vi "16ChannelRecorderv2.vi"() -> ()   [LabVIEW 2013]
doc: "Cont(inuous) Acq(uire) & Chart (hw timed) demonstrates the hardware timed, non-buffered technique of data acquisition. The scan clock on the board controls acquisition timing. Acquired scans are read directly from the device's FIFO using AI Single Scan. \n\nThe acquisition is configured with no buffer, and the on-board scan clock started at the selected scan rate. In the first loop iteration, the newest (most recent) scan is read from the FIFO. In each subsequent loop iteration AI Single Scan is called to read the oldest scan from the FIFO. Then if a scan is missed because the acquisition does not keep up, an error message will be displayed, and the acquisition stopped. Each scan is plotted on the chart after it is read. \n\nA common reason to use non-buffered acquisition is that some kind of processing needs to be done for each data point. You will probably want to add more functions to the diagram to customize this VI for your application. The acquisition rate you can achieve depends on how much processing and display the VI must do. This VI calls a subVI named My Single-Scan Processing. Add whatever processing you need to this subVI, or replace it with one of your own. The data processing subVI also demonstrates how to use error clusters in your own subVIs, so they can be included in the error data flow chain.\n\nBefore running this VI, set the values of the controls on the front panel. Select Show Help Window from the Help menu to see a description of each control. If the values you select for all the controls are values you will usually use, select Make Current Values Default from the Operate menu and save the VI. Or, you may save individual control's default values by popping up on the control, selecting Data Operations, then selecting Make Current Value Default, and saving the VI."
uses:
  <vilib>/Utility/error.llb/DialogType.ctl
  <vilib>/DAQmx/read.llb/DAQmx Read (Analog 2D DBL NChan NSamp).vi
  BiaxGlobals (16chan).vi
  <vilib>/DAQmx/create/channels.llb/DAQmx Create Channel (AI-Voltage-Basic).vi
  <vilib>/DAQmx/configure/timing.llb/DAQmx Timing (Sample Clock).vi
  effectiveglobals.vi
  <vilib>/DAQmx/miscellaneous.llb/DAQmx Fill In Error Info.vi
panel:
  in  "Show plot":bool
  out "Zero Voltage Y":dbl
  in  "Calibration y-axis (V/unit)":dbl=1.0 format="%#_6f"
  in  "Select y-axis":string(combo)="Porosity"
  in  "Calibration x-axis (V/unit)":dbl=1.0 format="%#_6f"
  in  "Select x-axis":string(combo)="Time (s)"
  out "Offset Voltage 2":dbl
  out "Offset Voltage 1":dbl
  in  "Offset X-axis 2":bool
  in  "Offset X-axis 1":bool
  in  "Zero y-axis":bool
  out "XY plot":cluster{"Y":dbl[], "Y":dbl[]}[](graph)
  in  "Reset plot":bool
  out "Zero Voltage X":dbl
  in  "Zero X-axis":bool
  out "Porosity (%)":dbl format="%_4f"
  in  "Material density (g/cm3)":dbl=2.17
  in  "Amount of material (g)":dbl=42.88 format="%_4f"
  in  "Thickness (2 layers, mm)":dbl=11.28 format="%_4f"
  in  "Zero Hor DCDT":bool
  out "Average Pore pressure":dbl=0.0015205308
  out "Zeroed at:":i32
  out "Zero Voltage":dbl format="%_6g"
  in  "Zero Pore pressure A":bool
  out "Zeroed at:":i32
  out "Zero Voltage":dbl format="%_6g"
  in  "Zero Pore pressure B":bool
  out "Effective normal \nstress (MPa)":dbl=0.0015205308
  in  "Sample\n Area (m2)":dbl=0.003078
  out "Zeroed at:":i32
  out "Zero Voltage":dbl format="%_6g"
  in  "Zero Confine":bool
  in  "Horizontal Load":bool=TRUE
  out "Zeroed at:":i32
  out "Zero Voltage":dbl format="%_6g"
  in  "Zero Normal":bool
  out "Array 2":i32[][](array[numeric])=[[10000, 0, -17, -1030, -696, -422, -1063, -1097, -410, -661, -1080]]
  out "AUX8 (ch11)":dbl format="%.4f"
  out "AUX7 (ch10)":dbl format="%.4f"
  out "AUX6 (ch9)":dbl format="%.4f"
  out "AUX5 (ch8)":dbl format="%.4f"
  out "AUX4 (ch7)":dbl format="%.4f"
  out "AUX3 (ch6)":dbl format="%.4f"
  out "AUX2 (ch5)":dbl format="%.4f"
  out "AUX1 (ch4)":dbl format="%.4f"
  out "Hor Load (ch0)":dbl format="%.4f"
  out "Vert Load (ch2)":dbl format="%.4f"
  out "Hor LVDT":dbl format="%.4f"
  out "Vert LVDT (ch3)":dbl format="%.4f"
  out "Array 17":i32[][](array[numeric])=[[10000, -673, -5, -1015, -683, -421, -1049, -1100, -413, -693, -1121]]
  out "Array 16":i32[][](array[numeric])=[[10000, -673, -5, -1015, -683, -421, -1049, -1100, -413, -693, -1121]]
  out "Array 15":i32[][](array[numeric])=[[10000, -673, -5, -1015, -683, -421, -1049, -1100, -413, -693, -1121]]
  out "Array 14":i32[][](array[numeric])=[[10000, -685, -5, -1012, -680, -418, -1052, -1092, -421, -673, -1097]]
  out "AUX12 (ch15)":dbl format="%.4f"
  out "AUX11 (ch14)":dbl format="%.4f"
  out "AUX10 (ch13)":dbl format="%.4f"
  out "AUX9 (ch12)":dbl format="%.4f"
  out "element 15":string
  out "element 14":string
  out "element 13":string
  out "element 12":string
  out "element 11":string
  out "element 10":string
  out "element 9":string
  out "element 8":string
  out "element 7":string
  out "element 6":string="  "
  out "element 5":string
  out "element 4":string
  out "element 3":string
  out "element 2":string
  out "element":string
  out "element":string
  out "Stress-strain-temp vs time (Voltage)":dbl[][](graph)
  out "Array 13":i32[][](array[numeric])
  out "Array 12":i32[][](array[numeric])
  out "Array 11":i32[][](array[numeric])
  out "Array 10":i32[][](array[numeric])
  out "Array 9":i32[][](array[numeric])
  out "Array 8":i32[][](array[numeric])
  out "Array 7":i32[][](array[numeric])
  out "Array 6":i32[][](array[numeric])
  out "Array 5":i32[][](array[numeric])
  out "Array 4":i32[][](array[numeric])
  out "Array 3":i32[][](array[numeric])
  out "Array":i32[][](array[numeric])
  out "10000":bool
  in  "10 kHz":bool
  out "Processor scan rate":i32
  out "Present sample number":i32
  in  "1 Hz":bool
  out "1":bool
  out "10":bool
  out "100":bool
  out "1000":bool
  in  "10 Hz":bool
  in  "100 Hz":bool
  in  "1000 Hz":bool
  out "Data Recording Rate":i32(slide) scale=1.0..10000.0
  out "Write interval":i32
  out "Write countdown":i32
  out "Time into data acq. (s)":i32
  out "Saved sample No.":i32
  out "Record rate (samp/s)":i32
  out "No. of scans in backlog":i32
  in  "stop":bool
  # "To File (24 bit)"
  # "Input Signals (volts)"
  # "S\nI\nG\nN\nA\nL\n\nV\nO\nL\nT\nA\nG\nE"
  # "Timestamp"
  # "Data Recording Info"
  # "Sample (point) Number"
  # "Acquisition Statistics"
  # "Low gain"
  # "High gain"
  # "NOTE:  This instrument will write data (time channel then Channels 0-15) to a user defined filename.  The file is written in binary format without a header. The time channel is comprised of numbers indicating the data recording frequency (eg 1, 10, 100, 1000, 10000  samples per second)."
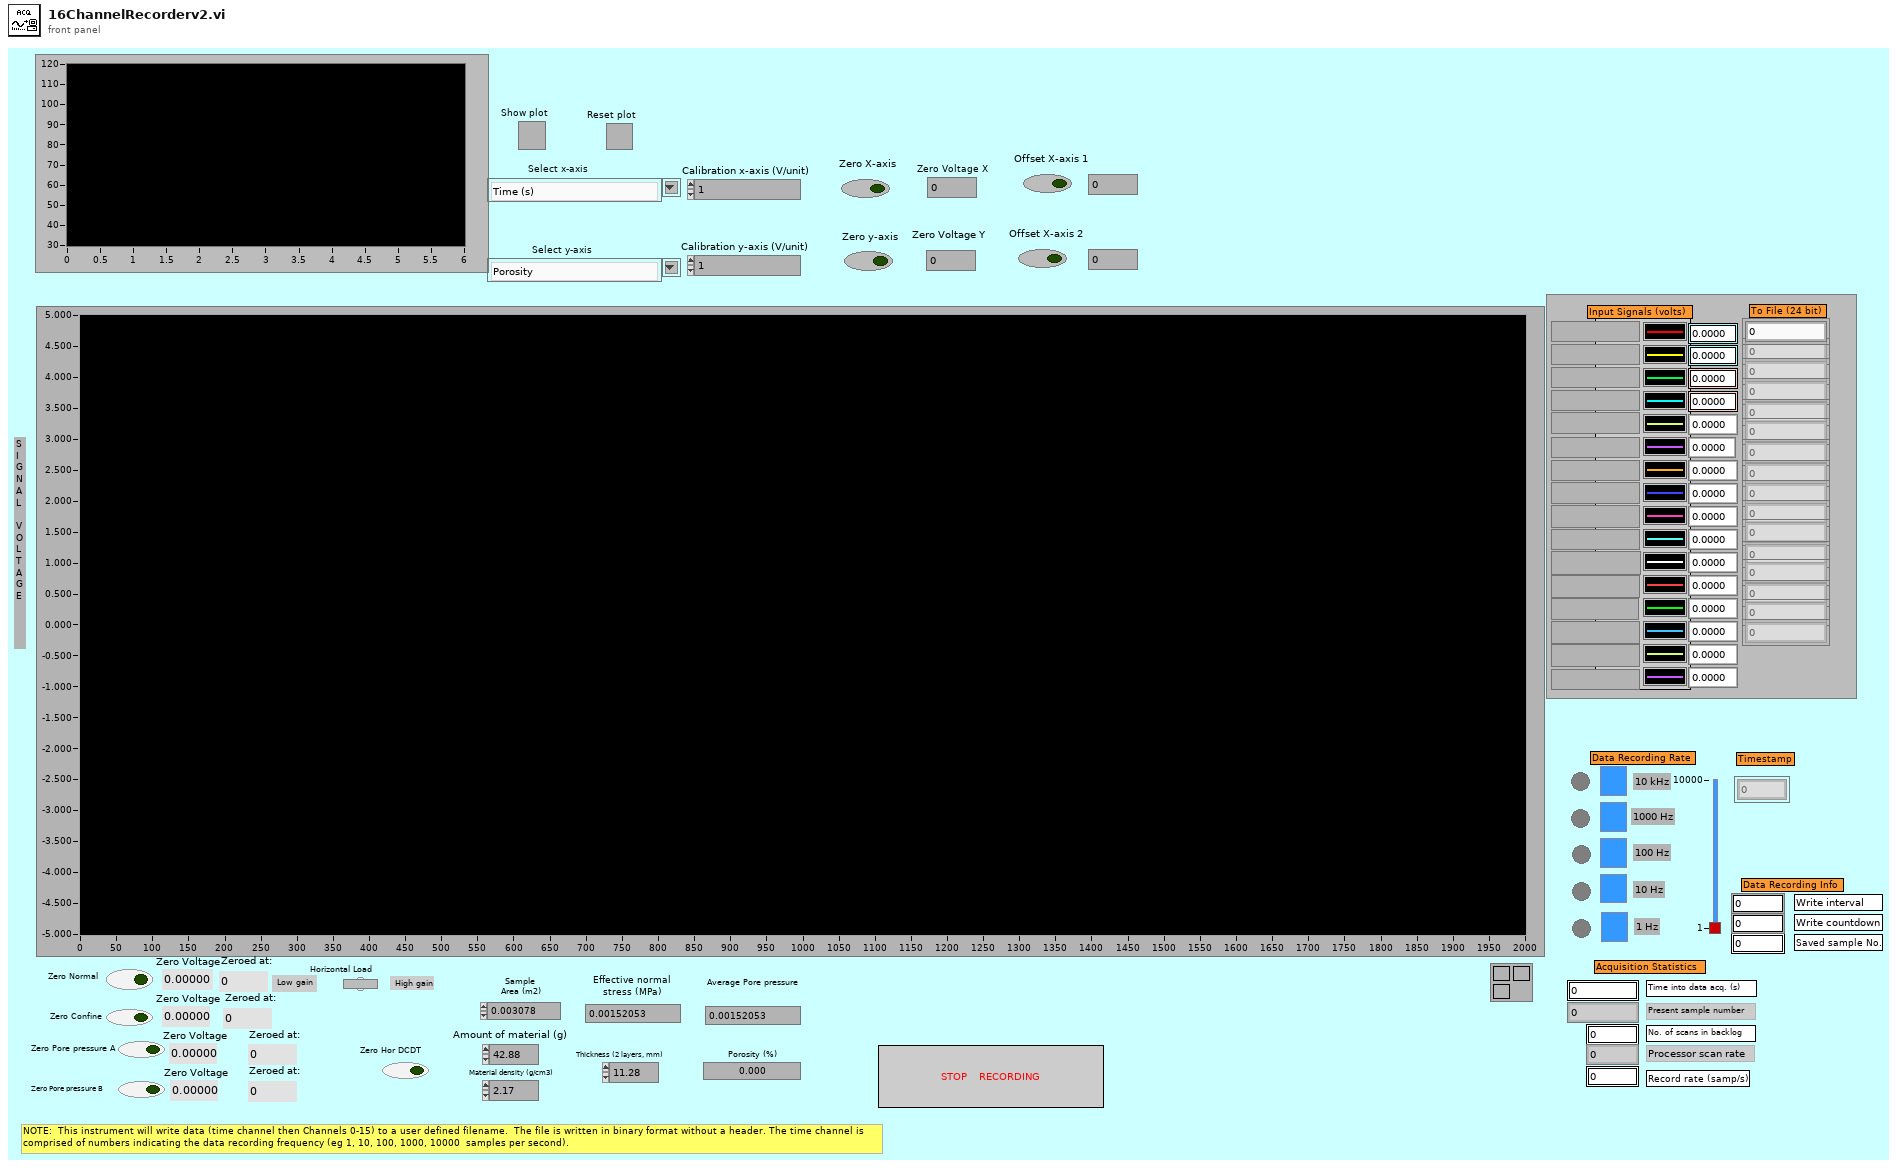
[diagram p1: front panel]
types:
  T1 = typedef "DialogType.ctl" = u16
  T2 = enum16{"big-endian, network order", "native, host order", "little-endian"}
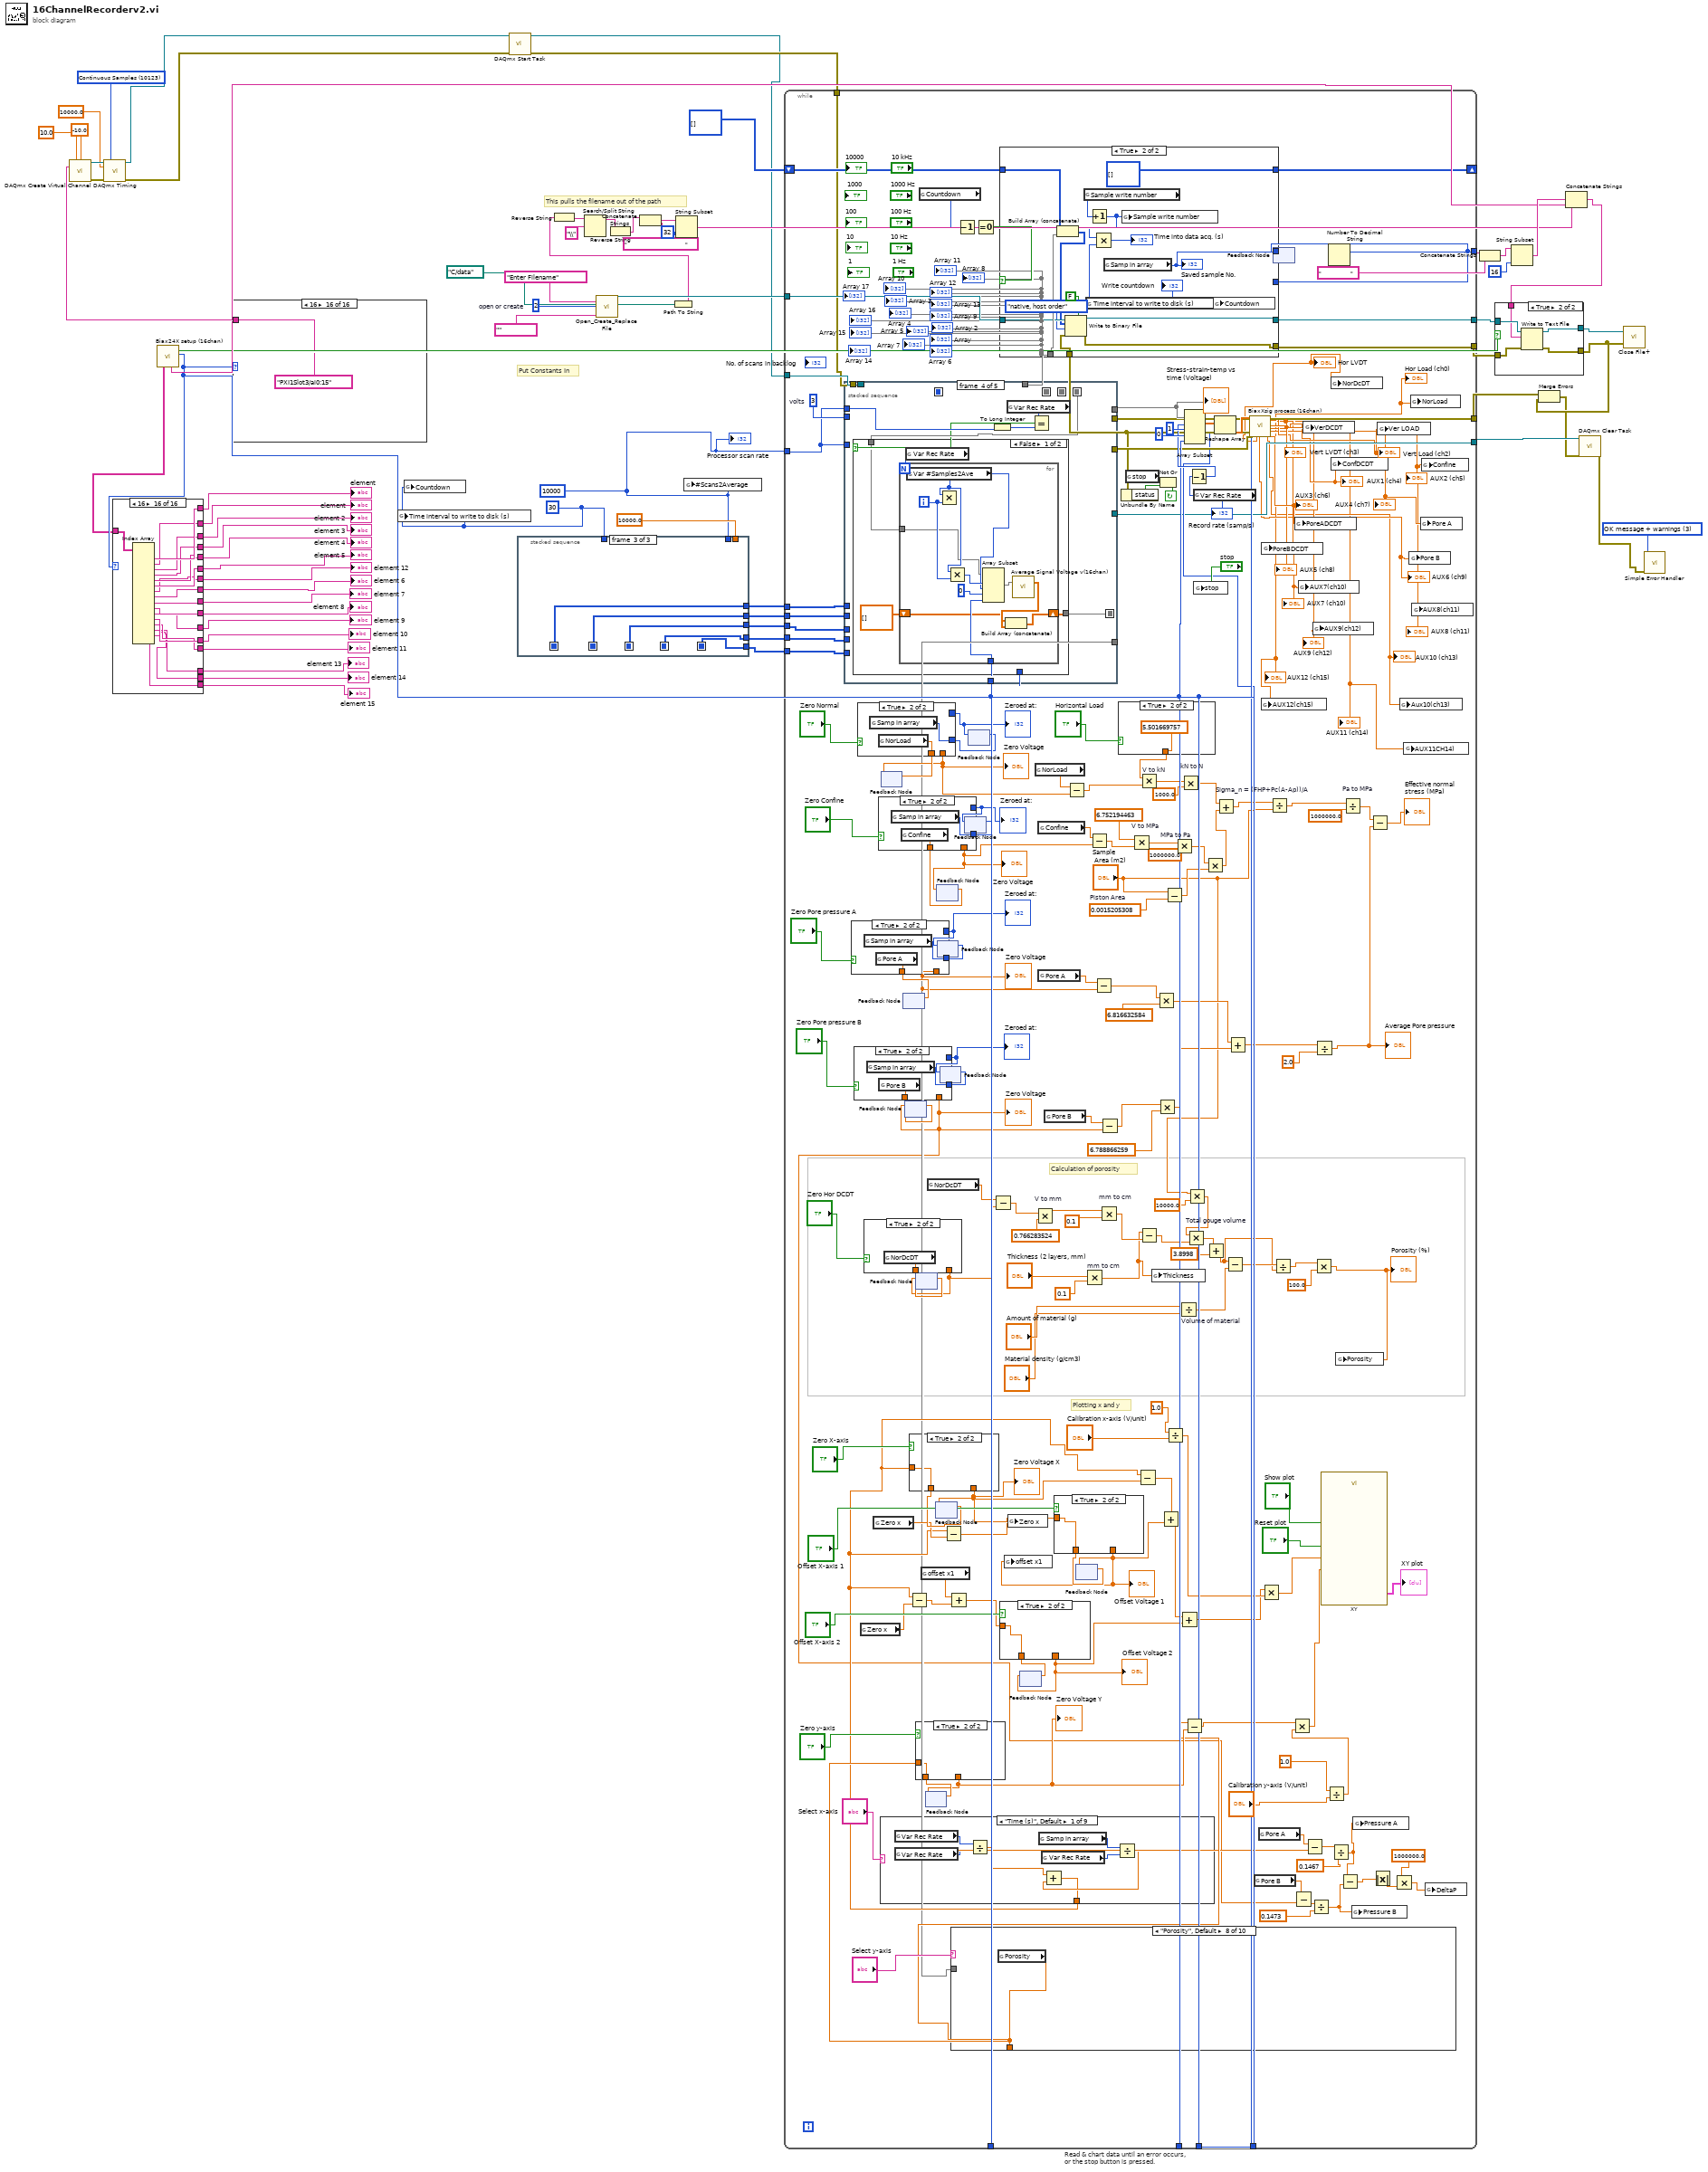
[diagram p0: block diagram]
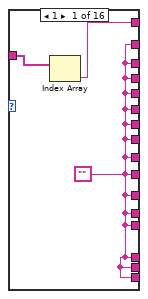
[diagram p2: hidden frame]
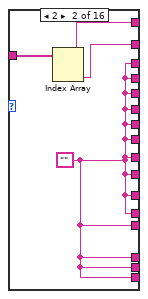
[diagram p3: hidden frame]
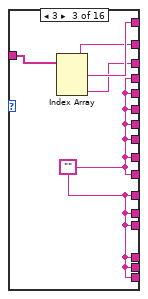
[diagram p4: hidden frame]
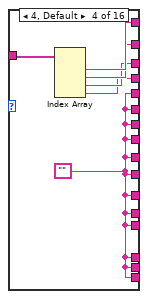
[diagram p5: hidden frame]
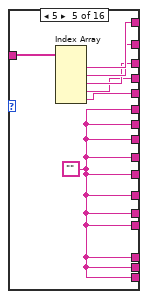
[diagram p6: hidden frame]
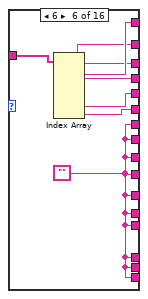
[diagram p7: hidden frame]
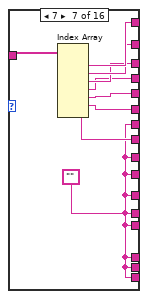
[diagram p8: hidden frame]
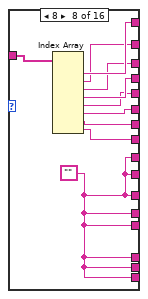
[diagram p9: hidden frame]
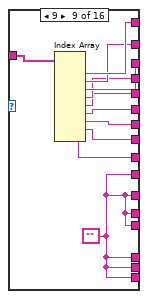
[diagram p10: hidden frame]
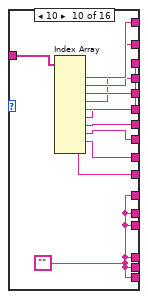
[diagram p11: hidden frame]
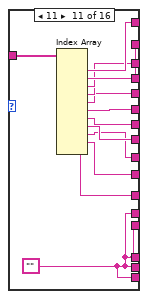
[diagram p12: hidden frame]
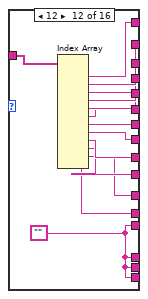
[diagram p13: hidden frame]
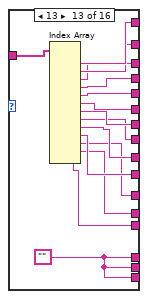
[diagram p14: hidden frame]
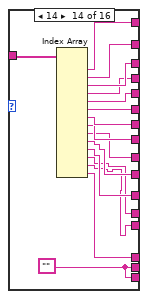
[diagram p15: hidden frame]
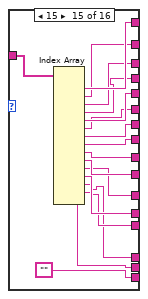
[diagram p16: hidden frame]
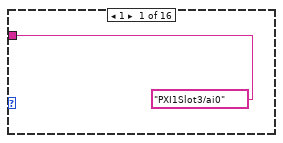
[diagram p18: hidden frame]
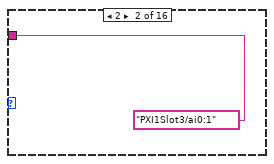
[diagram p19: hidden frame]
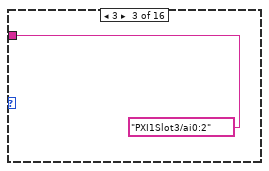
[diagram p20: hidden frame]
diagram:
  w11 = T1 3 items=["no dialog", "OK message", "continue or stop message", "OK message + warnings", "continue/stop + warnings"] ("type of dialog (OK msg:1)")
  w12 = 10000 ("Number of scans")
  w47 = 30 ("Write time int (s)")
  w50 = 10123 items=["Finite Samples"=10178, "Continuous Samples"=10123, "Hardware Timed Single Point"=12522] ("sample mode")
  w71 = 2  # open or create
  # "This pulls the filename out of the path"
  # "Put Constants In"
  n1 = call "Biax24X setup (16chan).vi"() -> ("Footer String"=w36:string, "Number of Channels"=w30:i32, "ASCII footer 2"=w35:bool, "Channel Names"=w29:string[])  [unwired: 1 in, 4 out]
  n2 = case shown="16" w30 {
    tunnel: w29 -> [w74 w77 w82 w88 w95 w103 w112 w123 w134 w146 w159 w173 w188 w202 w219 w238]
    tunnel: [w73 w78 w83 w89 w96 w104 w113 w122 w133 w145 w158 w172 w187 w201 w220 w237] -> w18
    tunnel: [w72 w76 w81 w87 w94 w102 w111 w121 w132 w144 w157 w171 w186 w200 w218 w236] -> w28
    tunnel: [w72 w75 w80 w86 w93 w101 w110 w120 w131 w143 w156 w170 w185 w199 w217 w235] -> w27
    tunnel: [w72 w75 w79 w85 w92 w100 w109 w119 w130 w142 w155 w169 w184 w198 w216 w234] -> w26
    tunnel: [w72 w75 w79 w84 w91 w99 w108 w118 w129 w141 w154 w168 w183 w197 w215 w233] -> w25
    tunnel: [w72 w75 w79 w84 w90 w98 w107 w117 w128 w140 w153 w167 w182 w196 w214 w232] -> w24
    tunnel: [w72 w75 w79 w84 w90 w97 w106 w115 w126 w138 w151 w165 w180 w194 w212 w230] -> w23
    tunnel: [w72 w75 w79 w84 w90 w97 w105 w114 w125 w137 w150 w164 w179 w193 w211 w229] -> w22
    tunnel: [w72 w75 w79 w84 w90 w97 w105 w114 w124 w136 w149 w163 w178 w191 w210 w228] -> w21
    tunnel: [w72 w75 w79 w84 w90 w97 w105 w114 w124 w135 w148 w162 w177 w192 w209 w227] -> w20
    tunnel: [w72 w75 w79 w84 w90 w97 w105 w114 w124 w135 w147 w161 w176 w190 w208 w226] -> w19
    tunnel: [w72 w75 w79 w84 w90 w97 w105 w114 w124 w135 w147 w160 w175 w189 w207 w225] -> w17
    tunnel: [w72 w75 w79 w84 w90 w97 w105 w114 w124 w135 w147 w160 w174 w203 w206 w224] -> w16
    tunnel: [w72 w75 w79 w84 w90 w97 w105 w114 w124 w135 w147 w160 w174 w204 w205 w223] -> w15
    tunnel: [w72 w75 w79 w84 w90 w97 w105 w114 w124 w135 w147 w160 w174 w204 "" w222] -> w14
    tunnel: [w72 w75 w79 w84 w90 w97 w105 w116 w127 w139 w152 w166 w181 w195 w213 w231] -> w13
    frame 1 {
      w72 = ""
      n3 = Index Array(array=w74) -> (element=w73:string)  [unwired: 1 in]
    }
    frame 2 {
      w75 = ""
      n4 = Index Array(array=w77) -> (element #1=w78:string, element #2=w76:string)  [unwired: 2 in]
    }
    frame 3 {
      w79 = ""
      n5 = Index Array(array=w82) -> (element #1=w83:string, element #2=w81:string, element #3=w80:string)  [unwired: 3 in]
    }
    frame 4, Default {
      w84 = ""
      n6 = Index Array(array=w88) -> (element #1=w89:string, element #2=w87:string, element #3=w86:string, element #4=w85:string)  [unwired: 4 in]
    }
    frame 5 {
      w90 = ""
      n7 = Index Array(array=w95) -> (element #1=w96:string, element #2=w94:string, element #3=w93:string, element #4=w92:string, element #5=w91:string)  [unwired: 5 in]
    }
    frame 6 {
      w97 = ""
      n8 = Index Array(array=w103) -> (element #1=w104:string, element #2=w102:string, element #3=w101:string, element #4=w100:string, element #5=w99:string, element #6=w98:string)  [unwired: 6 in]
    }
    frame 7 {
      w105 = ""
      n9 = Index Array(array=w112) -> (element #1=w113:string, element #2=w111:string, element #3=w110:string, element #4=w109:string, element #5=w108:string, element #6=w107:string, element #7=w106:string)  [unwired: 7 in]
    }
    frame 8 {
      w114 = ""
      n10 = Index Array(array=w123) -> (element #1=w122:string, element #2=w121:string, element #3=w120:string, element #4=w119:string, element #5=w118:string, element #6=w117:string, element #7=w116:string, element #8=w115:string)  [unwired: 8 in]
    }
    frame 9 {
      w124 = ""
      n11 = Index Array(array=w134) -> (element #1=w133:string, element #2=w132:string, element #3=w131:string, element #4=w130:string, element #5=w129:string, element #6=w128:string, element #7=w127:string, element #8=w126:string, element #9=w125:string)  [unwired: 9 in]
    }
    frame 10 {
      w135 = ""
      n12 = Index Array(array=w146) -> (element #1=w145:string, element #2=w144:string, element #3=w143:string, element #4=w142:string, element #5=w141:string, element #6=w140:string, element #7=w139:string, element #8=w138:string, element #9=w137:string, element #10=w136:string)  [unwired: 10 in]
    }
    frame 11 {
      w147 = ""
      n13 = Index Array(array=w159) -> (element #1=w158:string, element #2=w157:string, element #3=w156:string, element #4=w155:string, element #5=w154:string, element #6=w153:string, element #7=w152:string, element #8=w151:string, element #9=w150:string, element #10=w149:string, element #11=w148:string)  [unwired: 11 in]
    }
    frame 12 {
      w160 = ""
      n14 = Index Array(array=w173) -> (element #1=w172:string, element #2=w171:string, element #3=w170:string, element #4=w169:string, element #5=w168:string, element #6=w167:string, element #7=w166:string, element #8=w165:string, element #9=w164:string, element #10=w163:string, element #11=w162:string, element #12=w161:string)  [unwired: 12 in]
    }
    frame 13 {
      w174 = ""
      n15 = Index Array(array=w188) -> (element #1=w187:string, element #2=w186:string, element #3=w185:string, element #4=w184:string, element #5=w183:string, element #6=w182:string, element #7=w181:string, element #8=w180:string, element #9=w179:string, element #10=w178:string, element #11=w177:string, element #12=w176:string, element #13=w175:string)  [unwired: 13 in]
    }
    frame 14 {
      w204 = ""
      n16 = Index Array(array=w202) -> (element #1=w201:string, element #2=w200:string, element #3=w199:string, element #4=w198:string, element #5=w197:string, element #6=w196:string, element #7=w195:string, element #8=w194:string, element #9=w193:string, element #10=w191:string, element #11=w192:string, element #12=w190:string, element #13=w189:string, element #14=w203:string)  [unwired: 14 in]
    }
    frame 15 {
      n17 = Index Array(array=w219) -> (element #1=w220:string, element #2=w218:string, element #3=w217:string, element #4=w216:string, element #5=w215:string, element #6=w214:string, element #7=w213:string, element #8=w212:string, element #9=w211:string, element #10=w210:string, element #11=w209:string, element #12=w208:string, element #13=w207:string, element #14=w206:string, element #15=w205:string)  [unwired: 15 in]
    }
    frame 16 {
      n18 = Index Array(array=w238) -> (element #1=w237:string, element #2=w236:string, element #3=w235:string, element #4=w234:string, element #5=w233:string, element #6=w232:string, element #7=w231:string, element #8=w230:string, element #9=w229:string, element #10=w228:string, element #11=w227:string, element #12=w226:string, element #13=w225:string, element #14=w224:string, element #15=w223:string, element #16=w222:string)  [unwired: 16 in]
    }
  }
  "element" <- w18
  "element" <- w28
  "element 2" <- w27
  "element 3" <- w26
  "element 4" <- w25
  "element 5" <- w24
  "element 6" <- w23
  "element 7" <- w22
  "element 8" <- w21
  "element 9" <- w20
  "element 10" <- w19
  "element 11" <- w17
  "element 12" <- w13
  "element 13" <- w16
  "element 14" <- w15
  "element 15" <- w14
  n19 = case shown="16" w30 {
    tunnel: [tag "PXI1Slot3/ai0" ("physical channels") tag "PXI1Slot3/ai0:1" ("physical channels") tag "PXI1Slot3/ai0:2" ("physical channels") tag "PXI1Slot3/ai0:3" ("physical channels") tag "PXI1Slot3/ai0:4" ("physical channels") tag "PXI1Slot3/ai0:5" ("physical channels") tag "PXI1Slot3/ai0:6" ("physical channels") tag "PXI1Slot3/ai0:7" ("physical channels") tag "PXI1Slot3/ai0:8" ("physical channels") tag "PXI1Slot3/ai0:9" ("physical channels") tag "PXI1Slot3/ai0:10" ("physical channels") tag "PXI1Slot3/ai0:11" ("physical channels") tag "PXI1Slot3/ai0:12" ("physical channels") tag "PXI1Slot3/ai0:13" ("physical channels") tag "PXI1Slot3/ai0:14" ("physical channels") tag "PXI1Slot3/ai0:15" ("physical channels")] -> w44
    frame 1 {
    }
    frame 2 {
    }
    frame 3 {
    }
    frame 4, Default {
    }
    frame 5 {
    }
    frame 6 {
    }
    frame 7 {
    }
    frame 8 {
    }
    frame 9 {
    }
    frame 10 {
    }
    frame 11 {
    }
    frame 12 {
    }
    frame 13 {
    }
    frame 14 {
    }
    frame 15 {
    }
    frame 16 {
    }
  }
  n20 = call-poly <vilib>:"DAQmx Create Virtual Channel.vi"("maximum value"=10.0, "minimum value"=-10.0, "physical channels"=w44) -> ("task out"=w52:refnum<k21>, "error out"=w51:errorcluster)  [unwired: 11 in]
  n21 = call-poly <vilib>:"DAQmx Timing.vi"("task/channels in"=w52, "sample mode"=w50, "rate"=10000.0, "error in"=w51) -> ("task out"=w5:refnum<k21>, "error out"=w4:errorcluster)  [unwired: 10 in]
  n22 = global write "BiaxGlobals (16chan).vi" "Time interval to write to disk (s)"(w47) -> ()
  n23 = global write "BiaxGlobals (16chan).vi" "Countdown"(w47) -> ()
  n24 = call <vilib>:"DAQmx Start Task.vi"("task/channels in"=w5, "error in"=w4) -> ("task out"=w1:refnum<k21>, "error out"=w2:errorcluster)  [unwired: 12 in]
  n25 = stacked-sequence {
    seq-local: [_ w275 _] -> [_ _ w288]
    seq-local: [_ w272 _] -> [_ _ w285]
    seq-local: [_ w267 _] -> [_ _ w287]
    seq-local: [_ w266 _] -> [_ _ w286]
    seq-local: [_ w261 _] -> [_ _ w284]
    tunnel: w47 -> [w255 _ _]
    tunnel: w12 -> [w259 _ _]
    tunnel: sgl 10000.0 ("actual scan rate") -> [w257 _ _]
    tunnel: [_ _ w288] -> w66
    tunnel: [_ _ w285] -> w65
    tunnel: [_ _ w287] -> w64
    tunnel: [_ _ w286] -> w63
    tunnel: [_ _ w284] -> w62
    frame #0 {
      w256 = i16 0
      n26 = local write "Time into data acq. (s)"(w256) -> ()
      n27 = global write "BiaxGlobals (16chan).vi" "Sample write number"(w256) -> ()
      n28 = global write "BiaxGlobals (16chan).vi" "Time interval to write to disk (s)"(w255) -> ()
      n29 = Divide(x=w257, y=w259) -> (x/y=w258:sgl)
      n30 = global write "BiaxGlobals (16chan).vi" "Rec Rate (samp/s)"(w258) -> ()
      n31 = local write "Write countdown"(w255) -> ()
      n32 = local write "Saved sample No."(w256) -> ()
      n33 = global write "BiaxGlobals (16chan).vi" "Samp in array"(w256) -> ()
    }
    frame #1 {
      n34 = Initialize Array(i16 1, 10000) -> (w275:i16[])
      n35 = global write "BiaxGlobals (16chan).vi" "Rec Rate case"(4) -> ()
      n36 = local write "10"(FALSE) -> ()
      n37 = local write "1"(TRUE) -> ()
      n38 = Initialize Array(i16 10, 1000) -> (w272:i16[])
      n39 = local write "1000"(FALSE) -> ()
      n40 = local write "100"(FALSE) -> ()
      n41 = global read "BiaxGlobals (16chan).vi" "Time interval to write to disk (s)"() -> (→"Write interval":i32)
      n42 = Initialize Array(i16 100, 100) -> (w267:i16[])
      n43 = local write "10000"(FALSE) -> ()
      n44 = Initialize Array(i16 1000, 10) -> (w266:i16[])
      n45 = Initialize Array(i16 10000, 1) -> (w261:i16[])
      n46 = global write "BiaxGlobals (16chan).vi" "Accum Time"(0) -> ()
      n47 = global write "BiaxGlobals (16chan).vi" "Var Rec Rate"(1) -> ()
    }
    frame #2 {
    }
  }
  n48 = call <vilib>:"Open_Create_Replace File.vi"("default name"="", "prompt"="Enter Filename", "function (open:0)"=w71, "start path  (Not A Path)"=path "C:/data") -> ("new file path"=w61:path, "refnum"=w68:refnum<file>)  [unwired: 4 in, 2 out]
  n49 = Path To String(path=w61) -> (string=w58:string)
  n50 = Reverse String(1:w58) -> (0:w59:string)
  n51 = Search/Split String(string=w59, search string/char (-)="\\") -> (substring before match=w57:string)  [unwired: 1 in, 2 out]
  n52 = Reverse String(1:w57) -> (0:w53:string)
  n53 = Concatenate Strings(w53, "                                ") -> (w55:string)
  n54 = String Subset(string=w55, length (rest)=32 ("length (rest)")) -> (substring=w37:string)  [unwired: 1 in]
  n55 = global write "BiaxGlobals (16chan).vi" "#Scans2Average"(w12) -> ()
  n56 = while "Read & chart data until an error occurs,\nor the stop button is pressed." {
    tunnel: w62 -> [w450]
    tunnel: w63 -> [w452]
    tunnel: w64 -> [w453]
    tunnel: w65 -> [w454]
    tunnel: w66 -> [w455]
    shift-left: i16[][] [] -> [w442]
    shift-right: [w468] -> _
    tunnel: w12 -> [w456]
    tunnel: [w469] -> w32
    tunnel: [w470] -> w34
    tunnel: w68 -> [w471]
    tunnel: w30 -> [w449]
    tunnel: w30 -> [w443]
    tunnel: w30 -> [w448]
    tunnel: w30 -> [w444]
    tunnel: [w440] -> w43
    tunnel: w1 -> [w436]
    tunnel: w2 -> [w435]
    tunnel: [w434] -> w9
    tunnel: [w433] -> w10
    stop <- w467 continue-if-true
    w395 = 0.0015205308  # Piston Area
    w462 = 3  # volts
    # "Plotting x and y"
    # "Calculation of porosity"
    n57 = stacked-sequence {
      seq-local: [_ _ w587 _ _] -> [_ _ _ _ w629]
      seq-local: [_ _ _ w605 _] -> [_ _ _ _ w626]
      seq-local: [w551 _ _ _ _] -> [_ w556 _ _ _]
      seq-local: [_ w556 _ _ _] -> [_ _ w585 _ _]
      seq-local: [_ _ w585 _ _] -> [_ _ _ w604 _]
      tunnel: w462 -> [_ _ _ _ _]
      tunnel: w456 -> [_ _ _ w608 _]
      tunnel: [w549 _ _ _ _] -> w446
      tunnel: [_ _ _ _ w626] -> w439
      tunnel: w456 -> [w555 _ _ _ w634]
      tunnel: w455 -> [_ _ w595 _ _]
      tunnel: w454 -> [_ _ w594 _ _]
      tunnel: w453 -> [_ _ w593 _ _]
      tunnel: w452 -> [_ _ w592 _ _]
      tunnel: [_ _ _ _ w628] -> w437
      tunnel: w450 -> [_ _ w586 _ _]
      tunnel: w448 -> [_ _ _ w606 _]
      tunnel: w435 -> [w553 _ _ _ _]
      tunnel: w436 -> [w554 _ _ _ _]
      tunnel: [w549 _ _ _ _] -> w434
      tunnel: [w552 _ _ _ _] -> w433
      tunnel: [_ _ _ _ w626] -> w308
      frame #0 {
        n58 = call-poly <vilib>:"DAQmx Read.vi"("task/channels in"=w554, "number of samples per channel"=w555, "error in"=w553) -> ("task out"=w552:refnum<k21>, "data"=w550:dbl[][], "error out"=w549:errorcluster)  [unwired: 10 in]
        n59 = Transpose 2D Array(2D array=w550) -> (transposed array=w551:dbl[][])
      }
      frame #1 {
        n60 = local read "1000 Hz"() -> (w561:bool)
        n61 = local read "100 Hz"() -> (w560:bool)
        n62 = local read "10 Hz"() -> (w559:bool)
        n63 = local read "1 Hz"() -> (w558:bool)
        n64 = local read "10 kHz"() -> (w557:bool)
        n65 = case shown="True" w557 {
          frame False {
          }
          frame True {
            w562 = FALSE
            n66 = local write "1"(w562) -> ()
            n67 = local write "10"(w562) -> ()
            n68 = local write "100"(w562) -> ()
            n69 = local write "1000"(w562) -> ()
            n70 = local write "10000"(TRUE ("10x")) -> ()
            n71 = global write "BiaxGlobals (16chan).vi" "Rec Rate case"(0) -> ()
            n72 = global write "BiaxGlobals (16chan).vi" "Var Rec Rate"(10000) -> ()
          }
        }
        n73 = case shown="True" w561 {
          frame False {
          }
          frame True {
            w578 = FALSE
            n74 = local write "1"(w578) -> ()
            n75 = local write "10"(w578) -> ()
            n76 = local write "100"(w578) -> ()
            n77 = local write "10000"(w578) -> ()
            n78 = local write "1000"(TRUE ("10x")) -> ()
            n79 = global write "BiaxGlobals (16chan).vi" "Rec Rate case"(1) -> ()
            n80 = global write "BiaxGlobals (16chan).vi" "Var Rec Rate"(1000) -> ()
          }
        }
        n81 = case shown="True" w560 {
          frame False {
          }
          frame True {
            w574 = FALSE
            n82 = local write "1"(w574) -> ()
            n83 = local write "10"(w574) -> ()
            n84 = local write "1000"(w574) -> ()
            n85 = local write "10000"(w574) -> ()
            n86 = local write "100"(TRUE ("1x")) -> ()
            n87 = global write "BiaxGlobals (16chan).vi" "Rec Rate case"(2) -> ()
            n88 = global write "BiaxGlobals (16chan).vi" "Var Rec Rate"(100) -> ()
          }
        }
        n89 = case shown="True" w559 {
          frame False {
          }
          frame True {
            w570 = FALSE
            n90 = local write "1"(w570) -> ()
            n91 = local write "100"(w570) -> ()
            n92 = local write "1000"(w570) -> ()
            n93 = local write "10000"(w570) -> ()
            n94 = local write "10"(TRUE ("0.1x")) -> ()
            n95 = global write "BiaxGlobals (16chan).vi" "Rec Rate case"(3) -> ()
            n96 = global write "BiaxGlobals (16chan).vi" "Var Rec Rate"(10) -> ()
          }
        }
        n97 = case shown="True" w558 {
          frame False {
          }
          frame True {
            w566 = FALSE
            n98 = local write "10"(w566) -> ()
            n99 = local write "100"(w566) -> ()
            n100 = local write "1000"(w566) -> ()
            n101 = local write "10000"(w566) -> ()
            n102 = local write "1"(TRUE) -> ()
            n103 = global write "BiaxGlobals (16chan).vi" "Rec Rate case"(4) -> ()
            n104 = global write "BiaxGlobals (16chan).vi" "Var Rec Rate"(1) -> ()
          }
        }
      }
      frame #2 {
        n105 = global read "BiaxGlobals (16chan).vi" "Rec Rate case"() -> (w591:i32)
        n106 = case shown="1" w591 {
          tunnel: w595 -> [w598 _ _ _ _]
          tunnel: [w598 w599 w600 w601 w602] -> w587
          tunnel: w594 -> [_ w599 _ _ _]
          tunnel: w593 -> [_ _ w600 _ _]
          tunnel: w592 -> [_ _ _ w601 _]
          tunnel: w586 -> [_ _ _ _ w602]
          frame ..0 {
          }
          frame 1 {
          }
          frame 2 {
          }
          frame 3 {
          }
          frame 4.. {
          }
        }
        n107 = Array Size(array=w587) -> (size(s)=w590:i32)
        n108 = global read "BiaxGlobals (16chan).vi" "Countdown"() -> (w589:i32)
        n109 = global read "BiaxGlobals (16chan).vi" "Samp in array"() -> (w582:i32)
        n110 = global write "BiaxGlobals (16chan).vi" "Samp in array 0"(w582) -> ()
        n111 = Add(x=w582, y=w590) -> (x+y=w584:i32)
        "Present sample number" <- w584
        n112 = global read "BiaxGlobals (16chan).vi" "Var Rec Rate"() -> (w583:i32)
        "Data Recording Rate" <- w583
        n113 = global write "BiaxGlobals (16chan).vi" "Samp in array"(w584) -> ()
        n114 = global read "BiaxGlobals (16chan).vi" "#Scans2Average"() -> (w597:i16)
        n115 = Divide(x=w597, y=w583) -> (x/y=w596:dbl)
        n116 = Decrement(x=w589) -> (x-1=w588:i32)
        n117 = global write "BiaxGlobals (16chan).vi" "Var #Samples2Ave"(w596) -> ()
        n118 = local write "Write countdown"(w588) -> ()
      }
      frame #3 {
        n119 = To Long Integer(number=w608) -> (32bit integer=w607:i32)
        n120 = global read "BiaxGlobals (16chan).vi" "Var Rec Rate"() -> (w609:i32)
        n121 = Equal?(x=w609, y=w607) -> (x = y?=w603:bool)
        n122 = case shown="False" w603 {
          tunnel: w606 -> [w613 _]
          tunnel: w604 -> [w612 w625]
          tunnel: [w610 w625] -> w605
          frame False {
            n123 = global read "BiaxGlobals (16chan).vi" "Var Rec Rate"() -> (w614:i32)
            n124 = for {
              N: w614 -> [_]
              tunnel: w613 -> [w621]
              tunnel: w612 -> [w619]
              shift-right: [w615] -> w610
              shift-left: dbl[][] [] -> [w616]
              i -> [w624]
              n125 = global read "BiaxGlobals (16chan).vi" "Var #Samples2Ave"() -> (w620:i32)
              n126 = Multiply(x=w620, y=w624) -> ()  [unwired: 1 out]
              n127 = Multiply(x=w620, y=w624) -> (x*y=w622:i32)
              n128 = Array Subset(array=w619, index (row)=w622, length (row)=w620, index (col)=i16 0, length (col)=w621) -> (w618:dbl[][])
              n129 = call "Average Signal Voltage v(16chan).vi"("voltage data"=w618) -> ("average value\nper channel"=w617:dbl[])  [unwired: 2 in]
              n130 = Build Array (concatenate)(w616, w617) -> (w615:dbl[][])
            }
          }
          frame True {
          }
        }
      }
      frame #4 {
        (unwired) 1000.0
        n131 = global read "BiaxGlobals (16chan).vi" "Accum Time"() -> (w636:dbl)
        n132 = Transpose 2D Array(2D array=w626) -> (transposed array=w633:dbl[][])
        n133 = Multiply(x=838860.8, y=w633) -> (x*y=w631:dbl[][])
        n134 = To Long Integer(number=w631) -> (32bit integer=w630:i32[][])
        n135 = Add(x=w634, y=w636) -> (x+y=w635:dbl)
        n136 = Build Array (concatenate)(w629, w630) -> (w627:i32[][])
        n137 = Transpose 2D Array(2D array=w627) -> (transposed array=w628:i32[][])
        n138 = global write "BiaxGlobals (16chan).vi" "Accum Time"(w635) -> ()
      }
    }
    "Stress-strain-temp vs time (Voltage)" <- w439
    "Array" <- w437
    "Array 3" <- w437
    "Array 4" <- w437
    "Array 5" <- w437
    "Array 6" <- w437
    "Array 7" <- w437
    "Array 8" <- w437
    "Array 9" <- w437
    "Array 10" <- w437
    "Array 11" <- w437
    "Array 12" <- w437
    "Array 13" <- w437
    "Array 14" <- w437
    "Array 15" <- w437
    "Array 16" <- w437
    "Array 17" <- w437
    "Array 2" <- w437
    n139 = global read "effectiveglobals.vi" "Zero x"() -> (w312:dbl)
    n140 = global read "effectiveglobals.vi" "Zero x"() -> (w319:dbl)
    n141 = case shown="\"Time (s)\", Default" "Select x-axis" {
      tunnel: [w506 w513 w514 w515 w516 w517 w518 w519 w520] -> w313
      frame "Time (s)", Default {
        n142 = global read "BiaxGlobals (16chan).vi" "Var Rec Rate"() -> (w512:i32)
        n143 = global read "BiaxGlobals (16chan).vi" "Var Rec Rate"() -> (w511:i32)
        n144 = Divide(x=w512, y=w511) -> (x/y=w507:dbl)
        n145 = global read "BiaxGlobals (16chan).vi" "Samp in array"() -> (w510:i32)
        n146 = global read "BiaxGlobals (16chan).vi" "Var Rec Rate"() -> (w509:i32)
        n147 = Divide(x=w510, y=w509) -> (x/y=w508:dbl)
        n148 = Add(x=w507, y=w508) -> (x+y=w506:dbl)
      }
      frame "LP displacement" {
        n149 = global read "effectiveglobals.vi" "VerDCDT"() -> (w513:dbl)
      }
      frame "Shear load" {
        n150 = global read "effectiveglobals.vi" "Ver LOAD"() -> (w514:dbl)
      }
      frame "Normal displacement" {
        n151 = global read "effectiveglobals.vi" "NorDcDT"() -> (w515:dbl)
      }
      frame "Normal load" {
        n152 = global read "effectiveglobals.vi" "NorLoad"() -> (w516:dbl)
      }
      frame "Pore pressure A displacement" {
        n153 = global read "effectiveglobals.vi" "PoreADCDT"() -> (w517:dbl)
      }
      frame "Pore pressure A" {
        n154 = global read "effectiveglobals.vi" "Pore A"() -> (w518:dbl)
      }
      frame "Pore Preesure B Displacement" {
        n155 = global read "effectiveglobals.vi" "PoreBDCDT"() -> (w519:dbl)
      }
      frame "Pore Pressure B" {
        n156 = global read "effectiveglobals.vi" "Pore B"() -> (w520:dbl)
      }
    }
    n157 = feedback #1() -> (w411:dbl)  [unwired: 1 in]
    "Zero Voltage" <- w411
    n158 = feedback #2() -> (w293:dbl)  [unwired: 1 in]
    "Zero Voltage" <- w293
    n159 = feedback #3() -> (w292:dbl)  [unwired: 1 in]
    "Zero Voltage" <- w292
    n160 = Subtract(x=w313, y=w312) -> (x-y=w311:dbl)
    n161 = feedback #4() -> (w351:dbl)  [unwired: 1 in]
    n162 = case shown="True" "Zero Hor DCDT" {
      tunnel: [w529 w530] -> w364
      tunnel: w351 -> [w529 _]
      frame False {
      }
      frame True {
        n163 = global read "effectiveglobals.vi" "NorDcDT"() -> (w530:dbl)
      }
    }
    n164 = feedback-in #4(w364) -> ()
    n165 = global read "BiaxGlobals (16chan).vi" "Countdown"() -> (w451:i32)
    n166 = global read "effectiveglobals.vi" "offset x1"() -> (w310:dbl)
    n167 = feedback #5() -> (w327:dbl)  [unwired: 1 in]
    "Zero Voltage Y" <- w327
    n168 = global read "effectiveglobals.vi" "NorDcDT"() -> (w352:dbl)
    n169 = feedback #6() -> (w321:dbl)  [unwired: 1 in]
    "Zero Voltage X" <- w321
    n170 = case shown="True" "Zero X-axis" {
      tunnel: [w527 w528] -> w325
      tunnel: w313 -> [_ w528]
      tunnel: w321 -> [w527 _]
      frame False {
      }
      frame True {
      }
    }
    n171 = feedback-in #6(w325) -> ()
    n172 = feedback #7() -> (w401:dbl)  [unwired: 1 in]
    "Zero Voltage" <- w401
    n173 = feedback #8() -> (w384:i32)  [unwired: 1 in]
    "Zeroed at:" <- w384
    n174 = case shown="True" "Zero Pore pressure A" {
      tunnel: [w536 w538] -> w385
      tunnel: [w535 w537] -> w386
      tunnel: w293 -> [w535 _]
      tunnel: w384 -> [w536 _]
      frame False {
      }
      frame True {
        n175 = global read "BiaxGlobals (16chan).vi" "Samp in array"() -> (w538:i32)
        n176 = global read "effectiveglobals.vi" "Pore A"() -> (w537:dbl)
      }
    }
    n177 = feedback-in #2(w386) -> ()
    n178 = feedback-in #8(w385) -> ()
    n179 = feedback #9() -> (w381:i32)  [unwired: 1 in]
    "Zeroed at:" <- w381
    n180 = case shown="True" "Zero Pore pressure B" {
      tunnel: [w532 w534] -> w382
      tunnel: [w531 w533] -> w383
      tunnel: w292 -> [w531 _]
      tunnel: w381 -> [w532 _]
      frame False {
      }
      frame True {
        n181 = global read "BiaxGlobals (16chan).vi" "Samp in array"() -> (w534:i32)
        n182 = global read "effectiveglobals.vi" "Pore B"() -> (w533:dbl)
      }
    }
    n183 = feedback-in #3(w383) -> ()
    n184 = feedback-in #9(w382) -> ()
    n185 = Subtract(x=w313, y=w319) -> (x-y=w318:dbl)
    n186 = Add(x=w310, y=w311) -> (x+y=w309:dbl)
    n187 = case shown="\"Porosity\", Default" "Select y-axis" {
      tunnel: [w472 w473 w474 w475 w485 w501 w502 w503 w504 w505] -> w326
      tunnel: w308 -> [_ _ _ _ w494 _ _ _ _ _]
      frame "Shear load" {
        n188 = global read "effectiveglobals.vi" "Ver LOAD"() -> (w472:dbl)
      }
      frame "Normal displacement" {
        n189 = global read "effectiveglobals.vi" "NorDcDT"() -> (w473:dbl)
      }
      frame "Normal load" {
        n190 = global read "effectiveglobals.vi" "NorLoad"() -> (w474:dbl)
      }
      frame "Pore pressure A displacement" {
        n191 = global read "effectiveglobals.vi" "PoreADCDT"() -> (w475:dbl)
      }
      frame "Permeability A" {
        n192 = Array Subset(array=w494, index (row)=0 ("index"), length (row)=1 ("index")) -> (w499:dbl[][])  [unwired: 2 in]
        n193 = global read "BiaxGlobals (16chan).vi" "Samp in array"() -> (w496:i32)
        n194 = Reshape Array(w499, w496) -> (w497:dbl[])
        n195 = global read "effectiveglobals.vi" "PoreADCDT"() -> (w484:dbl)
        n196 = Index Array(array=w497, index=6) -> (element=w483:dbl)
        n197 = Subtract(x=w484, y=w483) -> (x-y=w479:dbl)
        n198 = Multiply(x=w479, y=0.025511) -> (x*y=w477:dbl)
        n199 = Absolute Value(x=w477) -> (abs(x)=w476:dbl)
        n200 = Multiply(x=0.005067074 ("y"), y=w476) -> (x*y=w490:dbl)
        n201 = global read "effectiveglobals.vi" "DeltaP"() -> (w487:dbl)
        n202 = Multiply(x=0.000889 ("y"), y=w490) -> (x*y=w492:dbl)
        n203 = global read "effectiveglobals.vi" "Thickness"() -> (w481:dbl)
        n204 = Multiply(x=w481, y=0.05) -> (x*y=w480:dbl)
        n205 = Multiply(x=w480, y=w492) -> (x*y=w489:dbl)
        n206 = Divide(x=w489, y=0.0049) -> (x/y=w486:dbl)
        n207 = Divide(x=w486, y=w487) -> (x/y=w485:dbl)
      }
      frame "Pore pressure A" {
        n208 = global read "effectiveglobals.vi" "Pressure A"() -> (w501:dbl)
      }
      frame "Pore pressure difference" {
        n209 = global read "effectiveglobals.vi" "DeltaP"() -> (w502:dbl)
      }
      frame "Porosity", Default {
        n210 = global read "effectiveglobals.vi" "Porosity"() -> (w503:dbl)
      }
      frame "Pore Pressure B displacement" {
        n211 = global read "effectiveglobals.vi" "PoreBDCDT"() -> (w504:dbl)
      }
      frame "Pore Pressure B" {
        n212 = global read "effectiveglobals.vi" "Pressure B"() -> (w505:dbl)
      }
    }
    n213 = case shown="True" "Zero y-axis" {
      tunnel: w326 -> [_ w526]
      tunnel: [w525 w526] -> w328
      tunnel: w327 -> [w525 _]
      frame False {
      }
      frame True {
      }
    }
    n214 = feedback-in #5(w328) -> ()
    n215 = Decrement(x=w451) -> (x-1=w438:i32)
    n216 = feedback #10() -> (w402:i32)  [unwired: 1 in]
    "Zeroed at:" <- w402
    n217 = case shown="True" "Zero Confine" {
      tunnel: [w540 w542] -> w403
      tunnel: [w539 w541] -> w404
      tunnel: w401 -> [w539 _]
      tunnel: w402 -> [w540 _]
      frame False {
      }
      frame True {
        n218 = global read "BiaxGlobals (16chan).vi" "Samp in array"() -> (w542:i32)
        n219 = global read "effectiveglobals.vi" "Confine"() -> (w541:dbl)
      }
    }
    n220 = feedback-in #7(w404) -> ()
    n221 = feedback-in #10(w403) -> ()
    n222 = feedback #11() -> (w413:i32)  [unwired: 1 in]
    "Zeroed at:" <- w413
    n223 = case shown="True" "Zero Normal" {
      tunnel: [w546 w548] -> w414
      tunnel: [w545 w547] -> w415
      tunnel: w411 -> [w545 _]
      tunnel: w413 -> [w546 _]
      frame False {
      }
      frame True {
        n224 = global read "BiaxGlobals (16chan).vi" "Samp in array"() -> (w548:i32)
        n225 = global read "effectiveglobals.vi" "NorLoad"() -> (w547:dbl)
      }
    }
    n226 = feedback-in #1(w415) -> ()
    n227 = feedback-in #11(w414) -> ()
    n228 = Equal To 0?(x=w438) -> (x = 0?=w463:bool)
    n229 = Subtract(x=w352, y=w351) -> (x-y=w350:dbl)
    n230 = global write "effectiveglobals.vi" "Zero x"(w321) -> ()
    n231 = feedback #12() -> (w316:dbl)  [unwired: 1 in]
    "Offset Voltage 2" <- w316
    n232 = case shown="True" "Offset X-axis 2" {
      tunnel: [w521 w522] -> w323
      tunnel: w316 -> [w521 _]
      tunnel: w309 -> [_ w522]
      frame False {
      }
      frame True {
      }
    }
    n233 = feedback-in #12(w323) -> ()
    n234 = global read "effectiveglobals.vi" "NorLoad"() -> (w410:dbl)
    n235 = Multiply "V to mm"(x=w350, y=0.766283524) -> (x*y=w363:dbl)
    n236 = global read "effectiveglobals.vi" "Confine"() -> (w400:dbl)
    n237 = global read "effectiveglobals.vi" "Pore A"() -> (w372:dbl)
    n238 = global read "effectiveglobals.vi" "Pore B"() -> (w369:dbl)
    n239 = Subtract(x=w410, y=w411) -> (x-y=w408:dbl)
    n240 = feedback #13() -> (w317:dbl)  [unwired: 1 in]
    "Offset Voltage 1" <- w317
    n241 = global write "effectiveglobals.vi" "offset x1"(w317) -> ()
    n242 = case shown="True" "Offset X-axis 1" {
      tunnel: [w523 w524] -> w320
      tunnel: w317 -> [w523 _]
      tunnel: w318 -> [_ w524]
      frame False {
      }
      frame True {
      }
    }
    n243 = feedback-in #13(w320) -> ()
    n244 = Multiply "mm to cm"(x="Thickness (2 layers, mm)", y=0.1 ("Thickness (2 layers, mm)")) -> (x*y=w306:dbl)
    n245 = Subtract(x=w400, y=w401) -> (x-y=w399:dbl)
    n246 = Subtract(x=w372, y=w293) -> (x-y=w371:dbl)
    n247 = Multiply "mm to cm"(x=w363, y=0.1) -> (x*y=w359:dbl)
    n248 = Subtract(x=w369, y=w292) -> (x-y=w368:dbl)
    n249 = case shown="True" "Horizontal Load" {
      tunnel: [52.91005291 5.501669757] -> w409
      frame False {
      }
      frame True {
      }
    }
    n250 = global read "BiaxGlobals (16chan).vi" "stop"() -> (w464:bool)
    n251 = Multiply "V to MPa"(x=6.752194463, y=w399) -> (x*y=w397:dbl)
    n252 = Subtract(x=w313, y=w321) -> (x-y=w339:dbl)
    n253 = Multiply "V to kN"(x=w409, y=w408) -> (x*y=w407:dbl)
    n254 = Subtract(x=w306, y=w359) -> (x-y=w346:dbl)
    n255 = global write "effectiveglobals.vi" "Thickness"(w306) -> ()
    n256 = Multiply(x=w371, y=6.816632584) -> (x*y=w370:dbl)
    n257 = Multiply(x=w368, y=6.788866259) -> (x*y=w367:dbl)
    n258 = Add(x=w339, y=w317) -> (x+y=w315:dbl)
    n259 = Subtract(x="Sample\n Area (m2)", y=w395) -> (x-y=w393:dbl)
    n260 = Divide(x=1.0, y="Calibration x-axis (V/unit)") -> (x/y=w334:dbl)
    n261 = Multiply "MPa to Pa"(x=w397, y=1000000.0) -> (x*y=w394:dbl)
    n262 = Divide "Volume of material"(x="Amount of material (g)", y="Material density (g/cm3)") -> (x/y=w356:dbl)
    n263 = Add(x=w315, y=w316) -> (x+y=w314:dbl)
    n264 = Multiply "kN to N"(x=w407, y=1000.0) -> (x*y=w392:dbl)
    n265 = Subtract(x=w326, y=w327) -> (x-y=w340:dbl)
    n266 = Multiply ("Total gouge volume")(x="Sample\n Area (m2)", y=10000.0) -> (x*y=w347:dbl)
    n267 = Multiply "Total gouge volume"(x=w347, y=w346) -> (x*y=w291:dbl)
    n268 = global read "BiaxGlobals (16chan).vi" "Var Rec Rate"() -> (w458:i32)
    "Record rate (samp/s)" <- w458
    n269 = Decrement(x=w458) -> (x-1=w457:i32)
    n270 = Array Subset(array=w439, index (row)=w457, length (row)=1, index (col)=0, length (col)=w449) -> (w460:dbl[][])
    n271 = global write "BiaxGlobals (16chan).vi" "stop"("stop") -> ()
    n272 = Multiply(x=w394, y=w393) -> (x*y=w391:dbl)
    n273 = Add(x=w291, y=3.8998) -> (x+y=w290:dbl)
    n274 = Reshape Array(w460, w443) -> (w447:dbl[])
    n275 = Add "Sigma_n = (FHP+Pc(A-Ap))/A"(x=w392, y=w391) -> (x+y=w390:dbl)
    n276 = Subtract(x=w290, y=w356) -> (x-y=w355:dbl)
    n277 = Add(x=w370, y=w367) -> (x+y=w378:dbl)
    n278 = call "BiaxXsig process (16chan).vi"("voltage data"=w447, "Numeric"=w444, "error in (no error)"=w446) -> ("AUX8"=w420:dbl, "AUX9"=w419:dbl, "Hor LVDT"=w430:dbl, "AUX7"=w421:dbl, "AUX6"=w422:dbl, "AUX5"=w423:dbl, "error out"=w445:errorcluster, "AUX12"=w418:dbl, "AUX4"=w424:dbl, "AUX11"=w416:dbl, "AUX10"=w417:dbl, "Hor Load"=w431:dbl, "Vert Load"=w428:dbl, "Ver LVDT"=w429:dbl, "AUX1"=w427:dbl, "AUX2"=w426:dbl, "AUX3"=w425:dbl)  [unwired: 7 in, 1 out]
    "Hor LVDT" <- w430
    "Hor Load (ch0)" <- w431
    "Vert Load (ch2)" <- w428
    "Vert LVDT (ch3)" <- w429
    "AUX1 (ch4)" <- w427
    "AUX2 (ch5)" <- w426
    "AUX3 (ch6)" <- w425
    "AUX4 (ch7)" <- w424
    "AUX5 (ch8)" <- w423
    "AUX6 (ch9)" <- w422
    "AUX7 (ch10)" <- w421
    "AUX8 (ch11)" <- w420
    "AUX9 (ch12)" <- w419
    "AUX10 (ch13)" <- w417
    "AUX11 (ch14)" <- w416
    "AUX12 (ch15)" <- w418
    n279 = Unbundle By Name(w445) -> ("status"=w466:bool)
    n280 = Not Or(1:w466, 2:w464) -> (0:w467:bool)
    n281 = global read "effectiveglobals.vi" "Pore B"() -> (w295:dbl)
    n282 = global read "effectiveglobals.vi" "Pore A"() -> (w300:dbl)
    n283 = Multiply(x=w314, y=w334) -> (x*y=w344:dbl)
    n284 = global write "effectiveglobals.vi" "AUX12(ch15)"(w418) -> ()
    n285 = global write "effectiveglobals.vi" "PoreBDCDT"(w423) -> ()
    n286 = Divide(x=w390, y="Sample\n Area (m2)") -> (x/y=w389:dbl)
    n287 = Divide ("material")(x=w355, y=w290) -> (x/y=w354:dbl)
    n288 = feedback #14() -> (w440:i32)  [unwired: 1 in]
    n289 = case shown="True" w463 {
      tunnel: w437 -> [w644 w654]
      tunnel: w442 -> [w643 w655]
      tunnel: w471 -> [w642 w651]
      tunnel: [w642 w650] -> w470
      tunnel: w445 -> [w641 w652]
      tunnel: [w641 w649] -> w469
      tunnel: [w638 i16[][] []] -> w468
      tunnel: [w637 w646] -> w441
      tunnel: w440 -> [w637 _]
      frame False {
        n290 = Build Array (concatenate)(w643, w644) -> (w638:i32[][])
        n291 = global read "BiaxGlobals (16chan).vi" "Countdown"() -> (w640:i32)
        n292 = Decrement(x=w640) -> (x-1=w639:i32)
        n293 = global write "BiaxGlobals (16chan).vi" "Countdown"(w639) -> ()
      }
      frame True {
        n294 = Build Array (concatenate)(w655, w654) -> (w648:i32[][])
        n295 = Write to Binary File(file (use dialog)=w651, data=w648, error in=w652, 5:FALSE ("prepend array or string size? (T)"), 9:T2."native, host order" ("byte order (0:big-endian, network order)")) -> (refnum out=w650:refnum<file>, error out=w649:errorcluster)  [unwired: 1 in, 1 out]
        n296 = global read "BiaxGlobals (16chan).vi" "Sample write number"() -> (w659:i16)
        n297 = global read "BiaxGlobals (16chan).vi" "Time interval to write to disk (s)"() -> (w656:i32)
        "Write countdown" <- w656
        n298 = Increment(x=w659) -> (x+1=w653:i16)
        n299 = Multiply(x=w653, y=w656) -> (x*y=→"Time into data acq. (s)":i32)
        n300 = global read "BiaxGlobals (16chan).vi" "Samp in array"() -> (w646:i32)
        "Saved sample No." <- w646
        n301 = global write "BiaxGlobals (16chan).vi" "Sample write number"(w653) -> ()
        n302 = global write "BiaxGlobals (16chan).vi" "Countdown"(w656) -> ()
      }
    }
    n303 = feedback-in #14(w441) -> ()
    n304 = Subtract(x=w295, y=w292) -> (x-y=w294:dbl)
    n305 = global write "effectiveglobals.vi" "PoreADCDT"(w425) -> ()
    n306 = global write "effectiveglobals.vi" "AUX7(ch10)"(w421) -> ()
    n307 = global write "effectiveglobals.vi" "VerDCDT"(w429) -> ()
    n308 = Subtract(x=w300, y=w293) -> (x-y=w299:dbl)
    n309 = Divide(x=w294, y=0.1473) -> (x/y=w296:dbl)
    n310 = global write "effectiveglobals.vi" "AUX9(ch12)"(w419) -> ()
    n311 = Multiply ("Total gouge volume")(x=w354, y=100.0 ("x*y")) -> (x*y=w322:dbl)
    "Porosity (%)" <- w322
    n312 = Divide(x=w378, y=2.0) -> (x/y=w374:dbl)
    "Average Pore pressure" <- w374
    n313 = Divide(x=1.0, y="Calibration y-axis (V/unit)") -> (x/y=w331:dbl)
    n314 = Multiply(x=w340, y=w331) -> (x*y=w307:dbl)
    n315 = call "XY.vi"("Enable"="Show plot", "Reset"="Reset plot", "Y Input"=w307, "X Input"=w344) -> ("XY Graph"=→"XY plot":cluster{"Y":dbl[], "Y":dbl[]}[])  [unwired: 6 in, 1 out]
    n316 = Divide(x=w299, y=0.1467) -> (x/y=w297:dbl)
    n317 = global write "effectiveglobals.vi" "NorDcDT"(w430) -> ()
    n318 = global write "effectiveglobals.vi" "ConfDCDT"(w427) -> ()
    n319 = global write "effectiveglobals.vi" "Porosity"(w322) -> ()
    n320 = Subtract(x=w297, y=w296) -> (x-y=w305:dbl)
    n321 = Divide "Pa to MPa"(x=w389, y=1000000.0) -> (x/y=w376:dbl)
    n322 = global write "effectiveglobals.vi" "Pressure B"(w296) -> ()
    n323 = global write "effectiveglobals.vi" "Pressure A"(w297) -> ()
    n324 = Subtract(x=w376, y=w374) -> (x-y=→"Effective normal \nstress (MPa)":dbl)
    n325 = Absolute Value(x=w305) -> (abs(x)=w304:dbl)
    n326 = global write "effectiveglobals.vi" "Ver LOAD"(w428) -> ()
    n327 = Multiply(x=1000000.0, y=w304) -> (x*y=w302:dbl)
    n328 = global write "effectiveglobals.vi" "Aux10(ch13)"(w417) -> ()
    n329 = global write "effectiveglobals.vi" "AUX11CH14)"(w416) -> ()
    n330 = global write "effectiveglobals.vi" "Pore B"(w422) -> ()
    n331 = global write "effectiveglobals.vi" "NorLoad"(w431) -> ()
    n332 = global write "effectiveglobals.vi" "AUX8(ch11)"(w420) -> ()
    n333 = global write "effectiveglobals.vi" "Pore A"(w424) -> ()
    n334 = global write "effectiveglobals.vi" "Confine"(w426) -> ()
    n335 = global write "effectiveglobals.vi" "DeltaP"(w302) -> ()
  }
  n336 = Number To Decimal String(number=w43) -> (decimal integer string=w42:string)  [unwired: 1 in]
  n337 = Concatenate Strings(w42, "                " ("string")) -> (w40:string)
  n338 = String Subset(string=w40, length (rest)=16 ("length (rest)")) -> (substring=w38:string)  [unwired: 1 in]
  n339 = Concatenate Strings(w37, w38, w36) -> (w31:string)
  n340 = case shown="True" w35 {
    tunnel: [w661 w665] -> w33
    tunnel: w34 -> [w661 w666]
    tunnel: w32 -> [w660 w663]
    tunnel: [w660 w664] -> w8
    tunnel: w31 -> [_ w662]
    frame False {
    }
    frame True {
      n341 = Write to Text File(file (use dialog)=w666, text=w662, error in=w663) -> (refnum out=w665:refnum<file>, error out=w664:errorcluster)  [unwired: 1 in, 1 out]
    }
  }
  n342 = Merge Errors(w9, w8) -> (w7:errorcluster)
  n343 = call <vilib>:"DAQmx Clear Task.vi"("task in"=w10, "error in"=w7) -> ("error out"=w3:errorcluster)  [unwired: 13 in]
  n344 = call <vilib>:"Close File+.vi"("error in (no error)"=w8, "refnum"=w33) -> ()  [unwired: 3 in, 3 out]
  n345 = call <vilib>:"Simple Error Handler.vi"("type of dialog (OK msg:1)"=w11, "error in (no error)"=w3) -> ()  [unwired: 3 in, 5 out]
  "Processor scan rate" <- w12
